vi "Write error for msg.vi"(8 "error in (no error)":errorcluster, 10 "error for msg":errorcluster, 11 "Error Display Actor in":refnum<class "Error Display Actor.lvclass">) -> (0 "error out":errorcluster, 3 "Error Display Actor out":refnum<class "Error Display Actor.lvclass">)   [LabVIEW 2020, in "ViewableActor.lvlib" / "Error Display Actor.lvclass"]
uses:
  Error Display Actor.lvclass
  Error Display Actor.lvclass/Error Display Actor.ctl
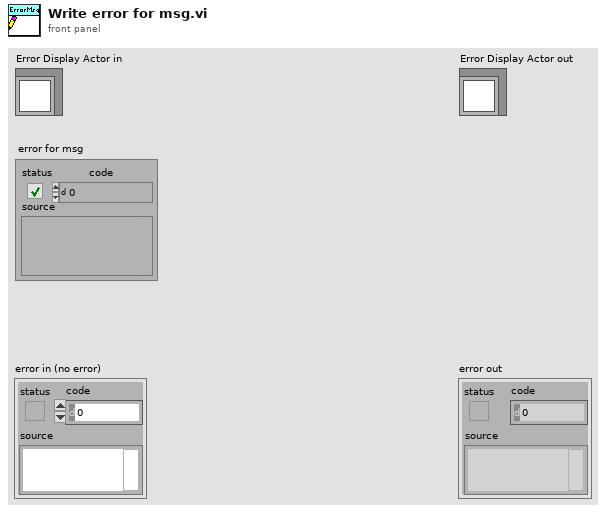
[diagram p1: front panel]
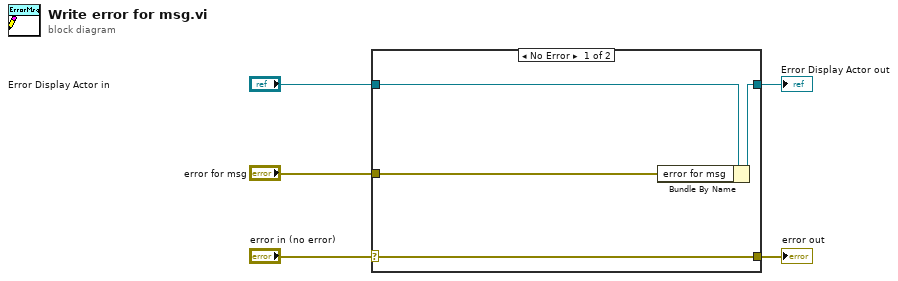
[diagram p0: block diagram]
diagram:
  n1 = case shown="No Error" "error in (no error)" {
    selector: "error in (no error)" -> [w9 w10]
    tunnel: [w9 w10] -> w4
    tunnel: [w7 w11] -> w2
    tunnel: "Error Display Actor in" -> [w8 w11]
    tunnel: "error for msg" -> [w6 _]
    frame No Error {
      n2 = Bundle By Name(cluster=w8, "error for msg"=w6) -> (w7:refnum<class "Error Display Actor.lvclass">)
    }
    frame Error {
    }
  }
  "error out" <- w4
  "Error Display Actor out" <- w2
